vi "dump analog buffer.vi"(5 "Relative Path Current Data":string, 6 "Date n Time":string, 7 "Base Path":path, 8 "error in":errorcluster, 9 "station idx":i32=4, 10 "ain buffer instead of motion buffer":bool, 11 "main state cluster":T1={"Application Status"="", "Switch Output Array"=[], "Switch Value Configuration"=[], "NVH Configuration"={"NVH Station?"=FALSE, "nvh app instance path"="", "NVH_ErrorMessages sv url"="", "NVH_Inputs sv url"="", "NVH_MotionNumber sv url"="", "NVH_Outputs sv url"="", "NVH_PartNumber sv url"="", "NVH_PartNumber_Echo sv url"="", "NVH_SerialNumber sv url"="", "NVH_AmbientTempF sv url"=""}, "rs232 port map"={"PMAC"="", "PS Port"="", "LVDT Unit"="", "RS232"=""}, "ethernet address map"={"LVDT 1 Unit"="172.17.53.143", "LVDT Unit 1 port"=0}, "paths"={"Base Path"=path "", "system error log path"=path "", "Error Table Path"=path "C/Labview Code/System/Error Table", "Store errors log path"=path "C/Labview Code/System/Error Table", "data bytes log path"=path "C/Labview Code/System/Error Table", "network path"=path "C/Labview Code/System/Error Table"}, "Station Index"=0, "Store Data"={"Motion Data Array"=[], "Error Table"=[], "Sun Shade Close Force Limits"={"Overall Min"=0.0, "Overall Max"=0.0, "Avg Min"=0.0, "Avg Max"=0.0, "Truncation Start"=0.0, "Truncation End"=0.0, "Variance"=0.0, "Check Noise"=FALSE}, "Sun Shade Open Force Limits"={"Overall Min"=0.0, "Overall Max"=0.0, "Avg Min"=0.0, "Avg Max"=0.0, "Truncation Start"=0.0, "Truncation End"=0.0, "Variance"=0.0, "Check Noise"=FALSE}, "Sunshade Open Data"=[], "Sunshade Close Data"=[], "Module Info"={"Serial Number"="", "Pallet Number"="", "Sunshade Color"="", "Inalfa Part Number"="", "Customer Number"=""}, "Sunsahde Close Raw Data"=[], "Sunshade Open Raw Data"=[], "Software Version"=[], "Constant Version"=[], "Hardware Version"=[], "Inalfa Part Number ECU"=[], "LVDT Data"=[], "Communication Line 1"=[], "Communication Line 2"=[], "Anti Pinch Force"=[], "Cycle Time"="", "Anti Pinch Vent Force"=[], "iGPS LVDT Data"=[], "data bytes log"=""}, "D in map"={"Abort Test"=enum."Dev2/port2/line6", "Start Test"=enum."Dev2/port2/line6"}, "DO Task"="", "ctl refs"={"Start Test"=refnum, "Abort Test"=refnum, "Manual Control"=refnum, "Route to Repair"=refnum, "Waveform Graph"=refnum, "Motion Data"=refnum, "all station status"=refnum, "Individual Station Status"=refnum, "exit program"=refnum, "Sunshade Servo Data Open"=refnum, "Sunshade Servo Data Close"=refnum, "Red-Rabbit Mode"=refnum, "Direct Manual Ctrl"=refnum}, "misc station config"={"Station Name"="", "is AT station?"=FALSE, "is audit station?"=FALSE, "power supply type"=enum."GENser", "use alt China TP2 LVDT Logic Seq"=FALSE, "hmi operator abort timeout"=0, "dump all analog values even if pass"=FALSE, "debug log pre-filter ap stream bytes"=FALSE, "use separate lvdt x and z extend tags"=FALSE, "is print"=FALSE}, "ethernet tcp refs"={"LVDT Unit"=refnum}, "Sunshade Barcode Scan"={"Sunshade Number 2"="", "Sunshade Number 1"="", "Keyence tuning bank idx"=0}, "AP Test Data"={"Raw Sunshade AP Data"="", "Raw Glass AP Data"="", "PMAC Read Counter"=0.0, "Database AP Data"=[]}, "Motion Status"={"hmi operator abort start time"=0, "Current Data Index"=0, "Analog Data"=[], "Motor Position Hex"=0, "Messages Index"=0, "Last Bytes"=[], "Current Hall Position"=0, "Motion Stop Timer"=0, "Position Test"=enum."Not Tested", "Noise Test"=enum."Not Tested", "motion stop check initialized"=FALSE, "remote sense enabled"=FALSE, "Motion"=enum."Glass Teach"}, "LVDT Status"={"LVDT's stored config"=[], "lvdt precision"={"truncate instead of rounding"=FALSE, "decimal places"=0}}, "Sequence State"={"Step Description"="", "Cycle Start Time"=0, "Step Data String"="", "Pass?"=FALSE, "Seqence"=[], "Active Step"=0, "Testing?"=FALSE, "Red-Rabbit Mode"=FALSE, "route-to-repair mode"=FALSE, "NVH Status"={"Restart IRQ Counter"=0, "NVH Test Needed?"=FALSE, "NVH Test Running?"=FALSE}, "Present (s)"=0.0, "Hold Mode?"=FALSE, "Hold?"=FALSE, "Rx Invalid?"=FALSE}, "misc status"={"delay start time (ticks)"=0, "In Vehicle Mode?"=FALSE, "Diag Mode?"=FALSE, "Serial Port Configured?"=FALSE, "PS Voltage"=0.0, "Diag Serial Port"="", "Part Setup"={"Communication Type"=enum."None", "Send Messages to"=enum."Glass", "RAP Signal"=enum."High", "Motor Type"=enum."Smart Motor", "NVH Part Number"=0, "Turn Off Timer"=0, "Part Type"=""}, "Part History Number"="", "Plant Number"=0, "AP Data Type"=enum."91/61", "Real Rollo?"=FALSE}, "NVH Operator?"=FALSE, "NVH Pass?"=FALSE, "Operator Pass?"=FALSE, "Operator Action?"=FALSE, "Noise Source"=0, "USBHandle"=0, "PeakInfo"="", "PeakNumber"=0, "NVH Motion Steps"=[], "Second Check?"=FALSE, "Decibel data"=[], "Direct Control Info"={"EnableStopOnHome"=FALSE, "EnableStopOnPos"=FALSE, "TeachEvent"=FALSE, "open offset"=0, "close offset"=0, "Derect control"=FALSE, "set position"=[], "teach pass "=FALSE, "Drift offsets"=[], "Hall Positions"=[]}, "manual control(direct)"=FALSE, "LIN INFO"={"Toolkit Type"=enum."Inalfa LIN", "NAD"=36, "Inalfa LIN"={"Master Frame(3C)"="", "Slave Frame(3D)"="NIXNET_exampleLDF", "Request Schedule"="NIXNET_exampleLDF", "Response Schedule"="CEMLIN3DiagResponseSchedule\nSPA3414_ConfigurationsCMAGeely_CEMCALYPSOSDB34XX0Cfg_LIN3_190709_", "Frame Write SCU"="", "Frame Read SCU"="", "LIN Name"=""}, "ADCS LIN"={"Port"="MasterReq\nSPA3414_ConfigurationsCMAGeely_CEMCALYPSOSDB34XX0Cfg_LIN3_190709_", "HW select"=0, "XNET Cluster"="SlaveResp\nSPA3414_ConfigurationsCMAGeely_CEMCALYPSOSDB34XX0Cfg_LIN3_190709_", "ByteCmd Path"=path "C/Labview Code/System/ByteCmdConfig.txt"}, "TS LIN"={"ref info"=refnum, "LIN Channel"=0, "ByteCmd Path"=path "C/Labview Code/System/ByteCmdConfig.txt"}}, "Config Info"=variant} {"LIN INFO"."NAD" format="%.0x"; "LIN INFO"."ADCS LIN"."HW select" items=["NI-XNET", "NI-CAN"]; "LVDT Status"."LVDT's stored config"."Lower Limit" format="%.2f"; "LVDT Status"."LVDT's stored config"."Upper Limit" format="%.2f"; "Store Data"."Sun Shade Open Force Limits"."Variance" format="%.2g"; "Store Data"."Sun Shade Open Force Limits"."Truncation End" format="%.2g"; "Store Data"."Sun Shade Open Force Limits"."Truncation Start" format="%.2g"; "Store Data"."Sun Shade Open Force Limits"."Avg Max" format="%.2g"; "Store Data"."Sun Shade Open Force Limits"."Avg Min" format="%.2g"; "Store Data"."Sun Shade Open Force Limits"."Overall Max" format="%.2g"; "Store Data"."Sun Shade Open Force Limits"."Overall Min" format="%.2g"; "Store Data"."Sun Shade Close Force Limits"."Variance" format="%.2g"; "Store Data"."Sun Shade Close Force Limits"."Truncation End" format="%.2g"; "Store Data"."Sun Shade Close Force Limits"."Truncation Start" format="%.2g"; "Store Data"."Sun Shade Close Force Limits"."Avg Max" format="%.2g"; "Store Data"."Sun Shade Close Force Limits"."Avg Min" format="%.2g"; "Store Data"."Sun Shade Close Force Limits"."Overall Max" format="%.2g"; "Store Data"."Sun Shade Close Force Limits"."Overall Min" format="%.2g"; "Store Data"."Motion Data Array"."Motion Data Limits"."LIN Msg"."Msg" format="%02x"; "Store Data"."Motion Data Array"."Motion Data Limits"."LIN Msg"."ID" format="%02x"}) -> (0 "error out":errorcluster)   [LabVIEW 2018]
uses:
  02.Type Def's/main state cluster.ctl
  02.Type Def's/All Switch Configuration Cluster.ctl
  02.Type Def's/All Motions.ctl
  02.Type Def's/EOL Switch Value Configuration Cluster.ctl
  02.Type Def's/EOL Switch Max Min Check Cluster.ctl
  02.Type Def's/station nvh config.ctl
  02.Type Def's/station rs232 port map.ctl
  02.Type Def's/station ethernet address map.ctl
  02.Type Def's/station paths.ctl
  02.Type Def's/EOL Save Module Test Data Control.ctl
  02.Type Def's/EOL Motion Database Table.ctl
  05.UserVI's/type defs/17x Audit Motion Data Seq Control.ctl
  05.UserVI's/type defs/17x AP Data Type.ctl
  05.UserVI's/type defs/17x Sunshade Limts Seq.ctl
  02.Type Def's/EOL Module Info Control.ctl
  02.Type Def's/station DI map.ctl
  05.UserVI's/type defs/EOL Global Digital Input Control.ctl
  02.Type Def's/control refs.ctl
  02.Type Def's/station motion data indicator.ctl
  02.Type Def's/Screen Motion Data.ctl
  02.Type Def's/Pass Fail Control.ctl
  02.Type Def's/station hmi.ctl
  02.Type Def's/lvdt name val pair.ctl
  02.Type Def's/individual station status.ctl
  02.Type Def's/misc station config.ctl
  05.UserVI's/Lambda Power/power supply types.ctl
  05.UserVI's/type defs/EOL LVDT's Check Controller.ctl
  05.UserVI's/LVDT's/lvdt precision.ctl
  02.Type Def's/sequence state.ctl
  05.UserVI's/sequence/type defs/Sequence Info.ctl
  05.UserVI's/type defs/EOL Part Setup.ctl
  02.Type Def's/All Communication Types.ctl
  05.UserVI's/type defs/Communication with Motors.ctl
  05.UserVI's/type defs/RAP Signal Control.ctl
  05.UserVI's/type defs/EOL Motor Type.ctl
  02.Type Def's/station LIN config.ctl
  03.Inalfa LIN/LIN Device.ctl
  <vilib>/CMC.AME/Inalfa ADCS/Ctl'Def/ADCS_LIN info.ctl
  C:/Program Files (x86)/National Instruments/LabVIEW 2018/vi.lib/CMC.AME/Inalfa TS LIN/TOSUN/TSMaster/bin/Interop.TSMasterAPI.dll
  Program Files (x86)/National Instruments/LabVIEW 2018/vi.lib/CMC.AME/Inalfa TS LIN/TOSUN/TSMaster/bin/Interop.TSMasterAPI.dll
  06.Test Loop/Sub'VIs/Type Def's/Config Info.ctl
panel:
  # "Sunroof Barcode"
  # "Pallet Number"
  # "Part Type"
  # "Application Status"
  # "Current Step"
  # "Cycle Time"
  # "Pass / Fail"
  # "Shade Close"
  # "Actual Data"
  # "Limits"
  # "Avg Current"
  # "Run Time"
  # "Speed"
  # "Noise Test"
  # "Position"
  # "Shade Open"
  # "Actual Data"
  # "Limits"
  # "Avg Current"
  # "Run Time"
  # "Speed"
  # "Noise Test"
  # "Position"
  # "Vent Close"
  # "Actual Data"
  # "Limits"
  # "Avg Current"
  # "Run Time"
  # "Speed"
  # "Noise Test"
  # "Position"
  # "Vent Open"
  # "Actual Data"
  # "Limits"
  # "Avg Current"
  # "Run Time"
  # "Speed"
  # "Noise Test"
  # "Position"
  # "Slide Close"
  # "Actual Data"
  # "Limits"
  # "Avg Current"
  # "Run Time"
  # "Speed"
  # "Noise Test"
  # "Position"
  # "Slide Open"
  # "Actual Data"
  # "Limits"
  # "Avg Current"
  # "Run Time"
  # "Speed"
  # "Noise Test"
  # "Position"
  # "Min"
  # "N"
  # "Min"
  # "Start"
  # "N"
  # "Max"
  # "N"
  # "Max"
  # "N"
  # "End"
  # "Min"
  # "N"
  # "Min"
  # "Start"
  # "N"
  # "Max"
  # "N"
  # "Max"
  # "N"
  # "End"
  # "Min"
  # "Max"
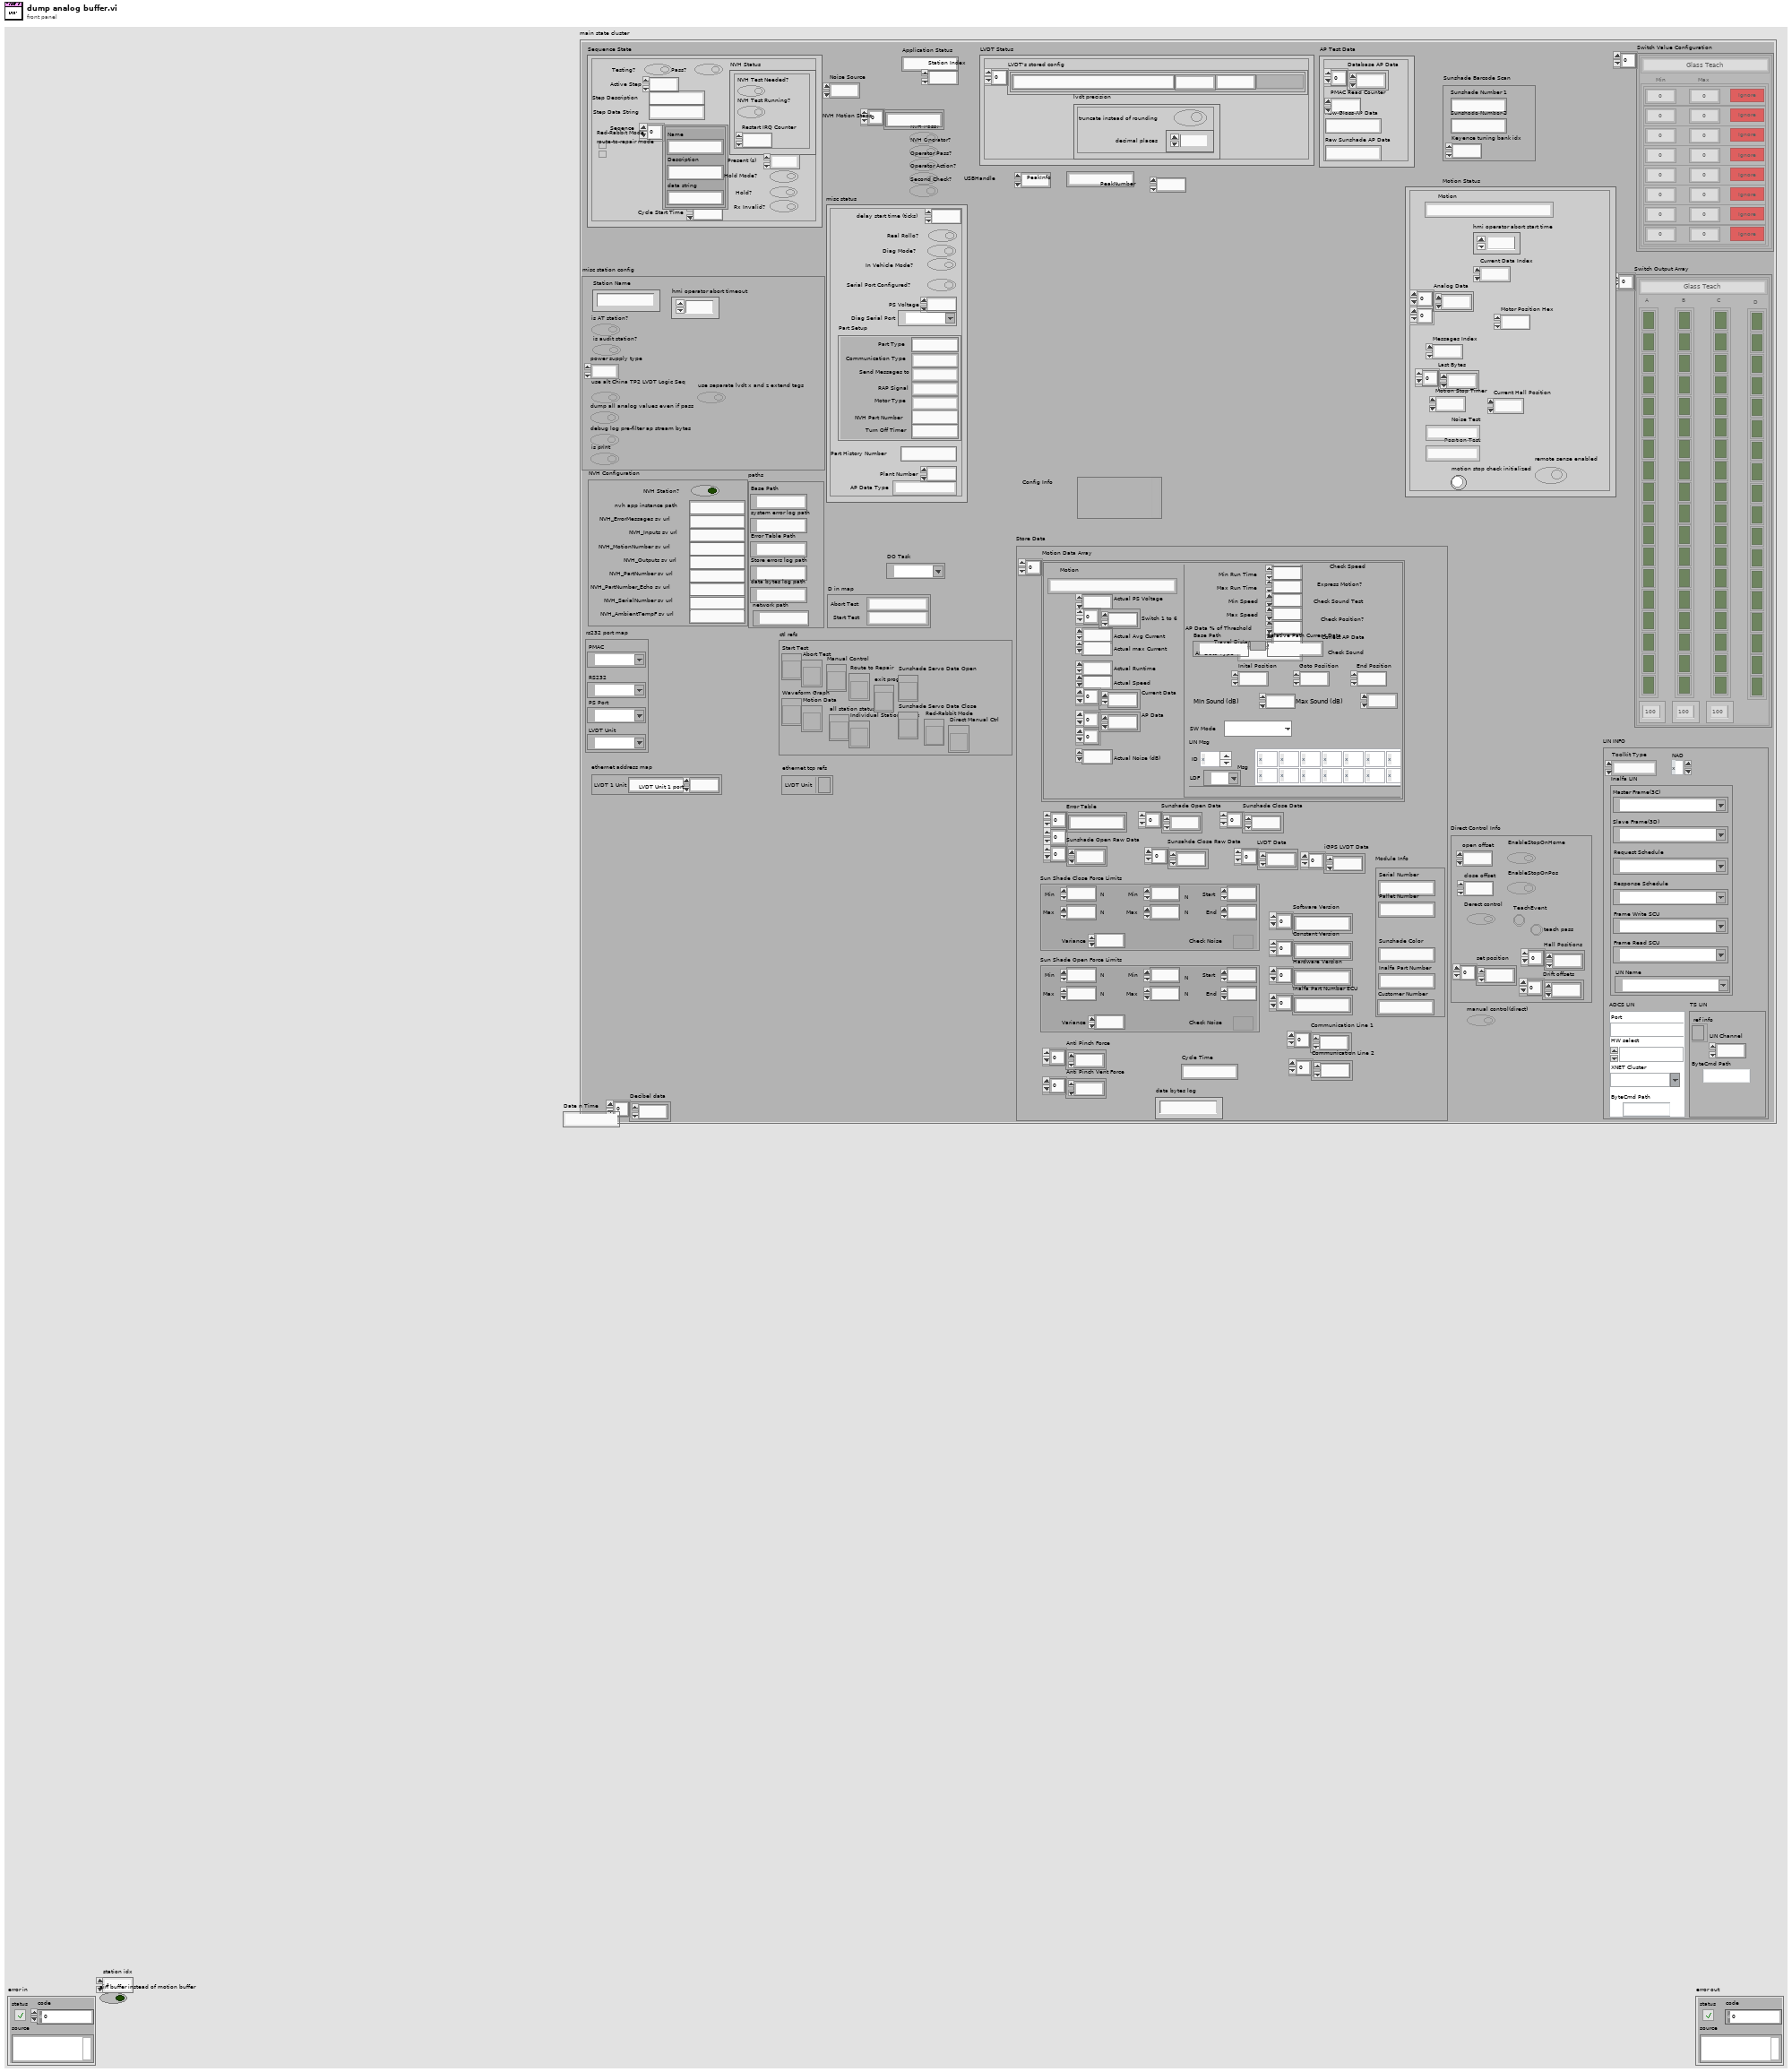
[diagram p1: front panel]
types:
  T1 = typedef "main state cluster.ctl" = cluster{"Application Status":string, "Switch Output Array":T2[], "Switch Value Configuration":T4[], "NVH Configuration":T6, "rs232 port map":T7, "ethernet address map":T8, "paths":T9, "Station Index":i32, "Store Data":T10, "D in map":T16, "DO Task":refnum<k21>, "ctl refs":T18, "misc station config":T19, "ethernet tcp refs":cluster{"LVDT Unit":refnum<k5>}, "Sunshade Barcode Scan":cluster{"Sunshade Number 2":string, "Sunshade Number 1":string, "Keyence tuning bank idx":i32}, "AP Test Data":cluster{"Raw Sunshade AP Data":string, "Raw Glass AP Data":string, "PMAC Read Counter":dbl, "Database AP Data":dbl[]}, "Motion Status":cluster{"hmi operator abort start time":u32, "Current Data Index":i32, "Analog Data":sgl[][], "Motor Position Hex":u16, "Messages Index":u16, "Last Bytes":u8[], "Current Hall Position":i16, "Motion Stop Timer":u32, "Position Test":T21, "Noise Test":T21, "motion stop check initialized":bool, "remote sense enabled":bool, "Motion":T3}, "LVDT Status":cluster{"LVDT's stored config":T22[], "lvdt precision":T23}, "Sequence State":T24, "misc status":cluster{"delay start time (ticks)":u32, "In Vehicle Mode?":bool, "Diag Mode?":bool, "Serial Port Configured?":bool, "PS Voltage":dbl, "Diag Serial Port":refnum<visa-resource-name>, "Part Setup":T26, "Part History Number":string, "Plant Number":u8, "AP Data Type":T13, "Real Rollo?":bool}, "NVH Operator?":bool, "NVH Pass?":bool, "Operator Pass?":bool, "Operator Action?":bool, "Noise Source":u32, "USBHandle":i32, "PeakInfo":string, "PeakNumber":i32, "NVH Motion Steps":string[], "Second Check?":bool, "Decibel data":dbl[], "Direct Control Info":cluster{"EnableStopOnHome":bool, "EnableStopOnPos":bool, "TeachEvent":bool, "open offset":i32, "close offset":i32, "Derect control":bool, "set position":i32[], "teach pass ":bool, "Drift offsets":i32[], "Hall Positions":i32[]}, "manual control(direct)":bool, "LIN INFO":T31, "Config Info":T34}
  T2 = typedef "All Switch Configuration Cluster.ctl" = cluster{"All Motions":T3, "A":bool[], "B":bool[], "C":bool[], "D":bool[], "A activation time (ms)":u32, "B activation time (ms)":u32, "C activation time (ms)":u32}
  T3 = typedef "All Motions.ctl" = enum16{"Glass Teach", "Glass Slide Open", "Glass Slide Close", "Glass Vent Open", "Glass Vent Close", "Sunshade Teach", "Sunshade Open", "Sunshade Close", "Idle", "Sunshade Open 2", "Sunshade Close 2", "Glass Slide Open Sunshade Open", "Glass Slide Open Sunshade Close", "Glass Slide Close Sunshade Open", "Glass Slide Close Sunshade Close", "Glass Vent Open Sunshade Open", "Glass Vent Open Sunshade Close", "Glass Vent Close Sunshade Open", "Glass Vent Close Sunshade Close", "Express Glass Slide Open", "Express Glass Slide Close", "Express Glass Vent Open", "Express Glass Vent Close", "Express Sunshade Open", "Express Sunshade Close", "Express Sunshade Open 2", "Express Sunshade Close 2", "Express Glass Slide Open Sunshade Open", "Express Glass Slide Open Sunshade Close", "Express Glass Slide Close Sunshade Open", "Express Glass Slide Close Sunshade Close", "Express Glass Vent Open Sunshade Open", "Express Glass Vent Open Sunshade Close", "Express Glass Vent Close Sunshade Open", "Express Glass Vent Close Sunshade Close", "Goto Position Glass", "Goto Position Sunshade", "Sunshade Teach 2"}
  T4 = typedef "EOL Switch Value Configuration Cluster.ctl" = cluster{"All Motions":T3, "Array":T5[]}
  T5 = typedef "EOL Switch Max Min Check Cluster.ctl" = cluster{"Min":dbl, "Max":dbl, "Check?":bool}
  T6 = typedef "station nvh config.ctl" = cluster{"NVH Station?":bool, "nvh app instance path":string, "NVH_ErrorMessages sv url":string, "NVH_Inputs sv url":string, "NVH_MotionNumber sv url":string, "NVH_Outputs sv url":string, "NVH_PartNumber sv url":string, "NVH_PartNumber_Echo sv url":string, "NVH_SerialNumber sv url":string, "NVH_AmbientTempF sv url":string}
  T7 = typedef "station rs232 port map.ctl" = cluster{"PMAC":refnum<visa-resource-name>, "PS Port":refnum<visa-resource-name>, "LVDT Unit":refnum<visa-resource-name>, "RS232":refnum<visa-resource-name>}
  T8 = typedef "station ethernet address map.ctl" = cluster{"LVDT 1 Unit":string, "LVDT Unit 1 port":u16}
  T9 = typedef "station paths.ctl" = cluster{"Base Path":path, "system error log path":path, "Error Table Path":path, "Store errors log path":path, "data bytes log path":path, "network path":path}
  T10 = typedef "EOL Save Module Test Data Control.ctl" = cluster{"Motion Data Array":T11[], "Error Table":string[][], "Sun Shade Close Force Limits":T14, "Sun Shade Open Force Limits":T14, "Sunshade Open Data":sgl[], "Sunshade Close Data":sgl[], "Module Info":T15, "Sunsahde Close Raw Data":sgl[], "Sunshade Open Raw Data":sgl[], "Software Version":string[], "Constant Version":string[], "Hardware Version":string[], "Inalfa Part Number ECU":string[], "LVDT Data":sgl[], "Communication Line 1":sgl[], "Communication Line 2":sgl[], "Anti Pinch Force":sgl[], "Cycle Time":string, "Anti Pinch Vent Force":sgl[], "iGPS LVDT Data":sgl[], "data bytes log":string}
  T11 = typedef "EOL Motion Database Table.ctl" = cluster{"Motion":T3, "Actual Avg Current":dbl, "Actual Runtime":dbl, "Actual Speed":dbl, "Current Data":sgl[], "Motion Data Limits":T12, "Switch 1 to 6":dbl[], "Actual PS Voltage":dbl, "AP Data":i16[][], "Actual max Current":dbl, "Actual Noise (dB)":dbl}
  T12 = typedef "17x Audit Motion Data Seq Control.ctl" = cluster{"Power Supply Voltage":dbl, "Min Avg Current":dbl, "Max Avg Current":dbl, "Min Run Time":dbl, "Max Run Time":dbl, "Min Speed":dbl, "Max Speed":dbl, "AP Data % of Threshold":dbl, "Travel Distance":dbl, "AP Data Type":T13, "Check Current":bool, "Check Run Time":bool, "Check Speed":bool, "Express Motion?":bool, "Check Sound Test":bool, "Check Position?":bool, "Collect AP Data":bool, "Inital Position":u16, "End Position":u16, "Goto Posiition":u16, "Max max Current":dbl, "Min max Current":dbl, "Check max Current":bool, "Check Sound":bool, "Min Sound (dB)":dbl, "Max Sound (dB)":dbl, "SW Mode":enum16{"Hard Switch", "Uncond Frame"}, "LIN Msg":cluster{"ID":u8, "Msg":u8[][], "LDF":refnum<k21>}}
  T13 = typedef "17x AP Data Type.ctl" = enum16{"91/61", "92/62", "93/63", "67", "68", "6F", "71", "91 Msg", "92 Msg", "93 Msg", "94 Msg", "HiRain 91", "HiRain 92 Speed", "HiRain 92 HS", "HiRain 92", "HiRain 93", "SnT"}
  T14 = typedef "17x Sunshade Limts Seq.ctl" = cluster{"Overall Min":dbl, "Overall Max":dbl, "Avg Min":dbl, "Avg Max":dbl, "Truncation Start":dbl, "Truncation End":dbl, "Variance":dbl, "Check Noise":bool}
  T15 = typedef "EOL Module Info Control.ctl" = cluster{"Serial Number":string, "Pallet Number":string, "Sunshade Color":string, "Inalfa Part Number":string, "Customer Number":string}
  T16 = typedef "station DI map.ctl" = cluster{"Abort Test":T17, "Start Test":T17}
  T17 = typedef "EOL Global Digital Input Control.ctl" = enum16{"Dev2/port0/line0", "Dev2/port0/line1", "Dev2/port0/line2", "Dev2/port0/line3", "Dev2/port0/line4", "Dev2/port0/line5", "Dev2/port0/line6", "Dev2/port0/line7", "Dev2/port1/line0", "Dev2/port1/line1", "Dev2/port1/line2", "Dev2/port1/line3", "Dev2/port1/line4", "Dev2/port1/line5", "Dev2/port1/line6", "Dev2/port1/line7", "Dev2/port2/line0", "Dev2/port2/line1", "Dev2/port2/line2", "Dev2/port2/line3", "Dev2/port2/line4", "Dev2/port2/line5", "Dev2/port2/line6", "Dev2/port2/line7", "Prerun Start Test", "Prerun Abort Test", "Audit Start Test", "Audit Abort Test", "Dev2/port3/line4", "Dev2/port3/line5", "Breakin Start Test", "Breakin Abort Test", "Not Implemented"}
  T18 = typedef "control refs.ctl" = cluster{"Start Test":refnum<vi>, "Abort Test":refnum<vi>, "Manual Control":refnum<vi>, "Route to Repair":refnum<vi>, "Waveform Graph":refnum<vi>, "Motion Data":refnum<vi>, "all station status":refnum<vi>, "Individual Station Status":refnum<vi>, "exit program":refnum<vi>, "Sunshade Servo Data Open":refnum<vi>, "Sunshade Servo Data Close":refnum<vi>, "Red-Rabbit Mode":refnum<vi>, "Direct Manual Ctrl":refnum<vi>}
  T19 = typedef "misc station config.ctl" = cluster{"Station Name":string, "is AT station?":bool, "is audit station?":bool, "power supply type":T20, "use alt China TP2 LVDT Logic Seq":bool, "hmi operator abort timeout":u32, "dump all analog values even if pass":bool, "debug log pre-filter ap stream bytes":bool, "use separate lvdt x and z extend tags":bool, "is print":bool}
  T20 = typedef "power supply types.ctl" = enum16{"GENser", "ZUPser", "GENeth", "Manual", "ITECH"}
  T21 = typedef "Pass Fail Control.ctl" = enum16{"Not Tested", "Pass", "Fail"}
  T22 = typedef "EOL LVDT's Check Controller.ctl" = cluster{"Upper Limit":dbl, "Lower Limit":dbl, "LVDT Name":string, "Check":bool}
  T23 = typedef "lvdt precision.ctl" = cluster{"truncate instead of rounding":bool, "decimal places":u8}
  T24 = typedef "sequence state.ctl" = cluster{"Step Description":string, "Cycle Start Time":u32, "Step Data String":string, "Pass?":bool, "Seqence":T25[], "Active Step":u8, "Testing?":bool, "Red-Rabbit Mode":bool, "route-to-repair mode":bool, "NVH Status":cluster{"Restart IRQ Counter":u8, "NVH Test Needed?":bool, "NVH Test Running?":bool}, "Present (s)":dbl, "Hold Mode?":bool, "Hold?":bool, "Rx Invalid?":bool}
  T25 = typedef "Sequence Info.ctl" = cluster{"Name":string, "Description":string, "data string":string}
  T26 = typedef "EOL Part Setup.ctl" = cluster{"Communication Type":T27, "Send Messages to":T28, "RAP Signal":T29, "Motor Type":T30, "NVH Part Number":u16, "Turn Off Timer":u16, "Part Type":string}
  T27 = typedef "All Communication Types.ctl" = enum16{"None", "CAN", "RS 232", "RS 232 LIN", "GM LIN", "SnT LIN", "K Line", "Robel CAN", "P42M-Continental", "Inalfa SCU LIN", "Spare 3"}
  T28 = typedef "Communication with Motors.ctl" = enum16{"Glass", "Rollo", "Both"}
  T29 = typedef "RAP Signal Control.ctl" = enum16{"High", "Low", "None"}
  T30 = typedef "EOL Motor Type.ctl" = enum16{"Smart Motor", "Sensor Motor"}
  T31 = typedef "station LIN config.ctl" = cluster{"Toolkit Type":enum16{"Inalfa LIN", "ADCS LIN", "TS LIN"}, "NAD":u8, "Inalfa LIN":T32, "ADCS LIN":T33, "TS LIN":cluster{"ref info":refnum<k24>, "LIN Channel":i32, "ByteCmd Path":path}}
  T32 = typedef "LIN Device.ctl" = cluster{"Master Frame(3C)":refnum<k21>, "Slave Frame(3D)":refnum<k21>, "Request Schedule":refnum<k21>, "Response Schedule":refnum<k21>, "Frame Write SCU":refnum<k21>, "Frame Read SCU":refnum<k21>, "LIN Name":refnum<k21>}
  T33 = typedef "ADCS_LIN info.ctl" = cluster{"Port":string, "HW select":u16, "XNET Cluster":string, "ByteCmd Path":path}
  T34 = typedef "Config Info.ctl" = variant
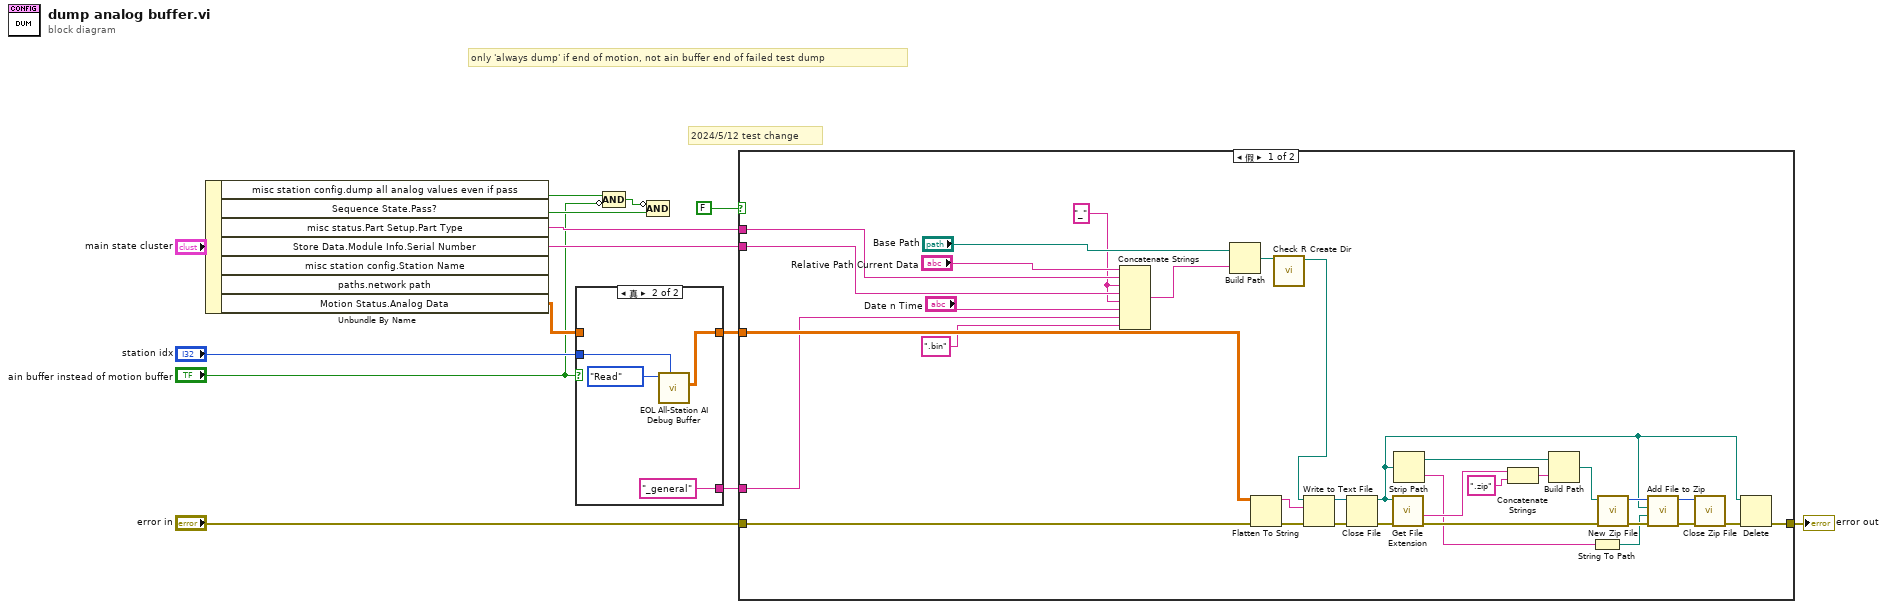
[diagram p0: block diagram]
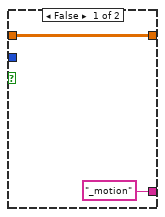
[diagram p2: hidden frame]
diagram:
  # "2024/5/12 test change"
  # "only 'always dump' if end of motion, not ain buffer end of failed test dump"
  n1 = Unbundle By Name("main state cluster") -> ("misc station config.dump all analog values even if pass"=w4:bool, "Sequence State.Pass?"=w10:bool, "misc status.Part Setup.Part Type"=w11:string, "Store Data.Module Info.Serial Number"=w12:string, "Motion Status.Analog Data"=w7:sgl[][])  [unwired: 2 out]
  n2 = case shown="真" "ain buffer instead of motion buffer" {
    tunnel: "station idx" -> [_ w18]
    tunnel: [w16 w17] -> w8
    tunnel: w7 -> [w16 _]
    tunnel: ["_motion" ("string") "_general" ("string")] -> w6
    frame False {
    }
    frame True {
      n3 = call "EOL All-Station AI Debug Buffer.vi"("station idx"=w18, "Mode"=enum16{"Initialize", "Read", "Write"}."Read") -> ("Data Read (Samp-Ro, Ch-Col)"=w17:sgl[][])  [unwired: 9 in]
    }
  }
  n4 = Compound Arithmetic op=AND(w4, invert "ain buffer instead of motion buffer") -> (w3:bool)
  n5 = Compound Arithmetic op=AND(invert w3, w10) -> ()  [unwired: 1 out]
  n6 = case shown="假" FALSE {
    tunnel: w8 -> [w52 _]
    tunnel: "error in" -> [w22 w54]
    tunnel: [w43 w54] -> w14
    tunnel: w12 -> [w27 _]
    tunnel: w11 -> [w28 _]
    tunnel: w6 -> [w26 _]
    frame False {
      w25 = "_" ("string")
      n7 = Concatenate Strings("Relative Path Current Data", w28, w25, w27, w25, "Date n Time", w26, ".bin" ("string")) -> (w30:string)
      n8 = Build Path(base path="Base Path", name or relative path=w30) -> (appended path=w29:path)
      n9 = Flatten To String(anything=w52, error in (no error)=w22) -> (data string=w53:string, error out=w51:errorcluster)  [unwired: 2 in, 1 out]
      n10 = call "Check R Create Dir.vi"("File Path"=w29) -> ("Dir Path"=w21:path)  [unwired: 10 in]
      n11 = Write to Text File(file (use dialog)=w21, text=w53, error in=w51) -> (refnum out=w46:refnum<file>, error out=w45:errorcluster)  [unwired: 1 in, 1 out]
      n12 = Close File(refnum=w46, error in=w45) -> (path=w35:path, error out=w42:errorcluster)
      n13 = call <vilib>:"Get File Extension.vi"("error in (no error)"=w42, "file"=w35) -> ("error out"=w37:errorcluster, "filename without extension"=w40:string)  [unwired: 5 in, 3 out]
      n14 = Strip Path(path=w35) -> (stripped path=w41:path, name=w34:string)
      n15 = Concatenate Strings(w40, ".zip" ("string")) -> (w36:string)
      n16 = Build Path(base path=w41, name or relative path=w36) -> (appended path=w38:path)
      n17 = String To Path(string=w34) -> (path=w33:path)
      n18 = call <vilib>:"New Zip File.vi"("error in (no error)"=w37, "target"=w38) -> ("error out"=w47:errorcluster, "zip file out"=w48:i64)  [unwired: 3 in, 1 out]
      n19 = call <vilib>:"Add File to Zip.vi"("error in (no error)"=w47, "destination path in zip"=w33, "source file path"=w35, "zip file in"=w48) -> ("error out"=w50:errorcluster, "zip file out"=w49:i64)  [unwired: 6 in]
      n20 = call <vilib>:"Close Zip File.vi"("error in (no error)"=w50, "zip file in"=w49) -> ("error out"=w44:errorcluster)  [unwired: 5 in]
      n21 = Delete(path (use dialog)=w35, error in=w44) -> (error out=w43:errorcluster)  [unwired: 3 in, 2 out]
    }
    frame True {
    }
  }
  "error out" <- w14
